vi "HEWH DO Nothing Condition.vi"(8 "error in (no error)":errorcluster, 10 "Saved Condition":T1, 11 "Current Cond":T1) -> (0 "error out":errorcluster, 3 "Current Cond Out":T1)   [LabVIEW 2020]
uses:
  Type Definitions/HEWH Special Condition Check.ctl
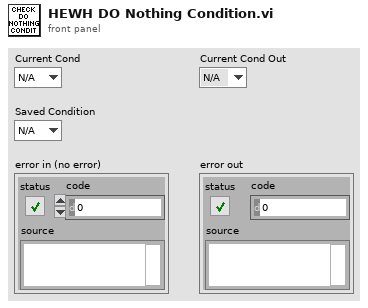
[diagram p1: front panel]
types:
  T1 = typedef "HEWH Special Condition Check.ctl" = enum16{"N/A", "C1", "C2", "Reset/Fail", "Skip Draw Sequence"}
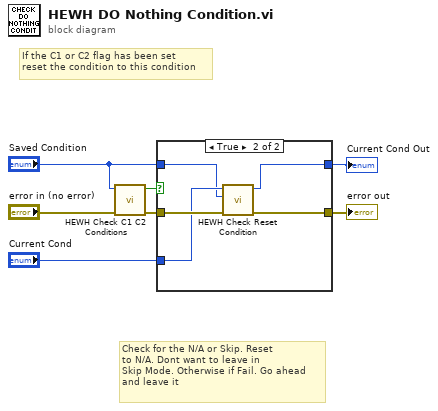
[diagram p0: block diagram]
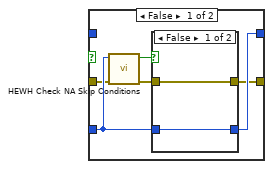
[diagram p2: hidden frame]
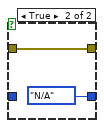
[diagram p3: hidden frame]
diagram:
  # "Check for the N/A or Skip. Reset\nto N/A. Dont want to leave in\nSkip Mode. Otherwise if Fail. Go ahead\nand leave it"
  # "If the C1 or C2 flag has been set\nreset the condition to this condition"
  n1 = call "HEWH Check C1 C2 Conditions.vi"("Error In"="error in (no error)", "Current Input"="Saved Condition") -> ("Error Out"=w2:errorcluster, "C1 or C2?"=w4:bool)  [unwired: 8 in]
  n2 = case shown="True" w4 {
    tunnel: "Saved Condition" -> [_ w19]
    tunnel: [w13 w18] -> w6
    tunnel: "Current Cond" -> [w11 w20]
    tunnel: w2 -> [w10 w22]
    tunnel: [w8 w21] -> w1
    frame False {
      n3 = call "HEWH Check NA Skip Conditions.vi"("Error In"=w10, "Current Input"=w11) -> ("Error Out"=w9:errorcluster, "N/A or Skip?"=w12:bool)  [unwired: 8 in]
      n4 = case shown="False" w12 {
        tunnel: [w15 HEWH_Special_Condition_Check."N/A" ("Saved Condition")] -> w13
        tunnel: w11 -> [w15 _]
        tunnel: [w14 w16] -> w8
        tunnel: w9 -> [w14 w16]
        frame False {
        }
        frame True {
        }
      }
    }
    frame True {
      n5 = call "HEWH Check Reset Condition.vi"("Error In"=w22, "SC3 Check Skip"=w19, "Current Cond"=w20) -> ("Error Out"=w21:errorcluster, "Current Cond"=w18:T1)  [unwired: 6 in, 1 out]
    }
  }
  "Current Cond Out" <- w6
  "error out" <- w1
